vi "SwissSPAD Live_Recording Message.vi"(8 "error in (no error)":errorcluster, 11 "SwissSPAD Live Internal Variables":T1={"okCFrontPanelDevices Refnum"=refnum, "Bottom Device Refnum"=refnum, "Display Image"=refnum, "# Live Images"=0, "relative s"=0.0, "# Image Sets"=0, "Message"="", "Current Image Set"=0, "# Datasets in Series"=0, "Current Dataset"=0, "Live Mode"=FALSE, "Recording Mode"=FALSE, "Record Button"=refnum, "\nLive Button"=refnum, "SwissSPAD Live Gate Image Data Q Name"="SS2 Live Gate Data Q", "Discard First Image"=FALSE, "Image Information"={"Save ROI Only"=FALSE, "Left"=0, "Top"=0, "Right"=0, "Bottom"=0, "Use Current ROI"=FALSE}, "Image Binning Options"={"Use Image Binning"=FALSE, "X Bin"=1, "Y Bin"=1}, "Bottom FPGA Serial Number"="", "Detector PCB Version"=enum."SS2 PCB1", "# Acquisitions"=1, "10 bits"=FALSE, "Top FPGA Serial Number"="", "Top Device Refnum"=refnum} {"# Acquisitions" min=1; "Image Binning Options"."Y Bin" min=1; "Image Binning Options"."X Bin" min=1}) -> (0 "error out":errorcluster, 1 "Current Dataset Recording Completed?":bool, 2 "Message":string, 3 "SwissSPAD Live Internal Variables":T1={"okCFrontPanelDevices Refnum"=refnum, "Bottom Device Refnum"=refnum, "Display Image"=refnum, "# Live Images"=0, "relative s"=0.0, "# Image Sets"=0, "Message"="", "Current Image Set"=0, "# Datasets in Series"=0, "Current Dataset"=0, "Live Mode"=FALSE, "Recording Mode"=FALSE, "Record Button"=refnum, "\nLive Button"=refnum, "SwissSPAD Live Gate Image Data Q Name"="SS2 Live Gate Data Q", "Discard First Image"=FALSE, "Image Information"={"Save ROI Only"=FALSE, "Left"=0, "Top"=0, "Right"=0, "Bottom"=0, "Use Current ROI"=FALSE}, "Image Binning Options"={"Use Image Binning"=FALSE, "X Bin"=1, "Y Bin"=1}, "Bottom FPGA Serial Number"="", "Detector PCB Version"=enum."SS2 PCB1", "# Acquisitions"=1, "10 bits"=FALSE, "Top FPGA Serial Number"="", "Top Device Refnum"=refnum} {"# Acquisitions" min=1; "Image Binning Options"."Y Bin" min=1; "Image Binning Options"."X Bin" min=1}, 4 "Dataset Series Completed?":bool)   [LabVIEW 2021]
uses:
  SwissSPAD Live_Internal Variables.ctl
  D:/UCLA Thinkpad Google Drive/LabVIEW 2021 SP1/builds/SwissSPAD Live Distribution/Opal Kelly/C# Wrapper/v5.0.2/libFrontPanel-csharp.dll
  Opal Kelly/C# Wrapper/v5.0.2/libFrontPanel-csharp.dll
  <vilib>/vision/Image Controls.llb/IMAQ Image.ctl
  SwissSPAD Live_Image ROI Information.ctl
  Phasor/Image Binning Options.ctl
  SwissSPAD Live_SSx PCB Version.ctl
  Sound/System Sounds List.ctl
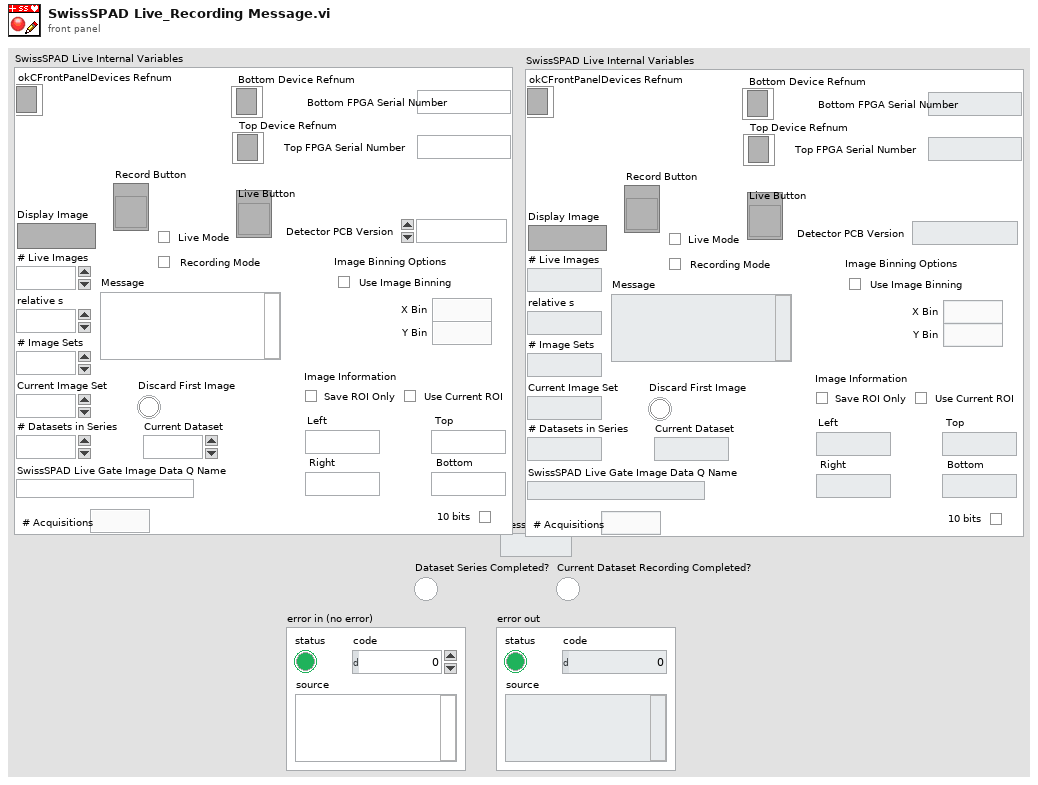
[diagram p1: front panel]
types:
  T1 = typedef "SwissSPAD Live_Internal Variables.ctl" = cluster{"okCFrontPanelDevices Refnum":refnum<k24>, "Bottom Device Refnum":refnum<k24>, "Display Image":T2, "# Live Images":i32, "relative s":dbl, "# Image Sets":i32, "Message":string, "Current Image Set":i32, "# Datasets in Series":i32, "Current Dataset":i32, "Live Mode":bool, "Recording Mode":bool, "Record Button":refnum<vi>, "\nLive Button":refnum<vi>, "SwissSPAD Live Gate Image Data Q Name":string, "Discard First Image":bool, "Image Information":T3, "Image Binning Options":T4, "Bottom FPGA Serial Number":string, "Detector PCB Version":T5, "# Acquisitions":u32, "10 bits":bool, "Top FPGA Serial Number":string, "Top Device Refnum":refnum<k24>}
  T2 = typedef "IMAQ Image.ctl" = refnum<image>
  T3 = typedef "SwissSPAD Live_Image ROI Information.ctl" = cluster{"Save ROI Only":bool, "Left":u16, "Top":u16, "Right":u16, "Bottom":u16, "Use Current ROI":bool}
  T4 = typedef "Image Binning Options.ctl" = cluster{"Use Image Binning":bool, "X Bin":i32, "Y Bin":i32}
  T5 = typedef "SwissSPAD Live_SSx PCB Version.ctl" = enum16{"unknown", "SS2 PCB1", "SS2 PCB2", "SS3 PCB1"}
  T6 = typedef "System Sounds List.ctl" = enum16{"Alarm01", "Alarm02", "Alarm03", "Alarm04", "Alarm05", "Alarm06", "Alarm07", "Alarm08", "Alarm09", "Alarm10", "chimes", "chord", "ding", "notify", "recycle", "Ring01", "Ring02", "Ring03", "Ring04", "Ring05", "Ring06", "Ring07", "Ring08", "Ring09", "Ring10", "ringout", "Speech Off", "Speech On", "Speech Sleep", "tada", "Windows Background", "Windows Balloon", "Windows Battery Critical", "Windows Battery Low", "Windows Critical Stop", "Windows Default", "Windows Ding", "Windows Error", "Windows Exclamation", "Windows Feed Discovered", "Windows Foreground", "Windows Hardware Fail", "Windows Hardware Insert", "Windows Hardware Remove", "Windows Information Bar", "Windows Logoff Sound", "Windows Logon", "Windows Menu Command", "Windows Message Nudge", "Windows Minimize", "Windows Navigation Start", "Windows Notify Calendar", "Windows Notify Email", "Windows Notify Messaging", "Windows Notify System Generic", "Windows Notify", "Windows Pop-up Blocked", "Windows Print complete", "Windows Proximity Connection", "Windows Proximity Notification", "Windows Recycle", "Windows Restore", "Windows Ringin", "Windows Ringout", "Windows Shutdown", "Windows Startup", "Windows Unlock", "Windows User Account Control"}
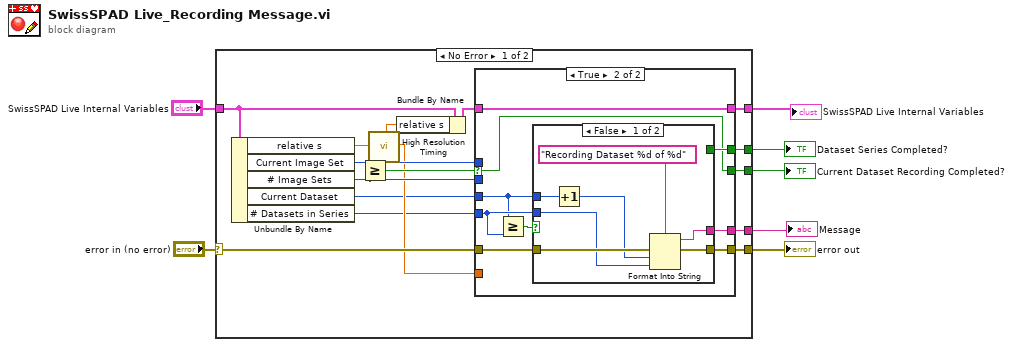
[diagram p0: block diagram]
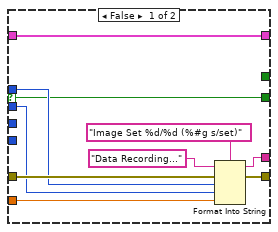
[diagram p2: hidden frame]
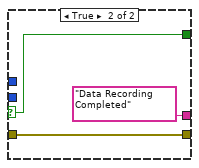
[diagram p3: hidden frame]
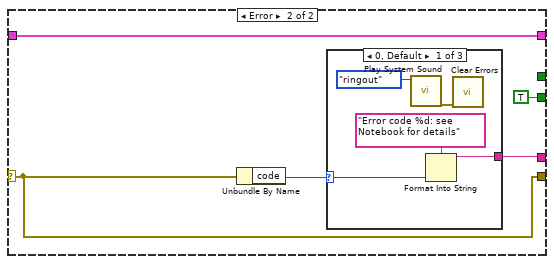
[diagram p4: hidden frame]
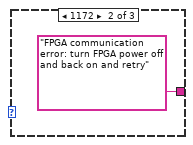
[diagram p5: hidden frame]
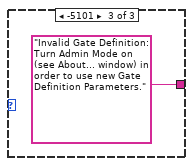
[diagram p6: hidden frame]
diagram:
  n1 = case shown="No Error" "error in (no error)" {
    selector: "error in (no error)" -> [w22 w55]
    tunnel: [w23 w55] -> w7
    tunnel: [w21 w56] -> w5
    tunnel: "SwissSPAD Live Internal Variables" -> [w20 w54]
    tunnel: [w9 w54] -> w3
    tunnel: [w11 TRUE] -> w2
    tunnel: [w8 _] -> w1
    frame No Error {
      n2 = Unbundle By Name(w20) -> ("relative s"=w16:dbl, "Current Image Set"=w18:i32, "# Image Sets"=w17:i32, "Current Dataset"=w13:i32, "# Datasets in Series"=w14:i32)
      n3 = Greater Or Equal?(x=w18, y=w17) -> (x >= y?=w19:bool)
      n4 = call "High Resolution Timing.vi"("relative seconds (NaN)"=w16) -> ("relative seconds"=w12:dbl, "elapsed (relative) seconds"=w15:dbl)  [unwired: 16 in, 1 out]
      n5 = Bundle By Name(cluster=w20, "relative s"=w12) -> (w10:T1)
      n6 = case shown="True" w19 {
        selector: w19 -> [w25 w34]
        tunnel: [w32 w41] -> w23
        tunnel: w22 -> [w31 w42]
        tunnel: [w30 w40] -> w21
        tunnel: w18 -> [w27 _]
        tunnel: w17 -> [w28 _]
        tunnel: w15 -> [w26 _]
        tunnel: w14 -> [_ w38]
        tunnel: w13 -> [_ w35]
        tunnel: [w25 w34] -> w11
        tunnel: w10 -> [w24 w36]
        tunnel: [w24 w36] -> w9
        tunnel: [_ w37] -> w8
        frame False {
          n7 = Format Into String(format string="Image Set %d/%d (%#g s/set)", initial string="Data Recording..." ("Message"), error in=w31, w27, w28, w26) -> (resulting string=w30:string, error out=w32:errorcluster)
        }
        frame True {
          n8 = Greater Or Equal?(x=w35, y=w38) -> (x >= y?=w39:bool)
          n9 = case shown="False" w39 {
            selector: w39 -> [_ w50]
            tunnel: w42 -> [w49 w51]
            tunnel: [w48 w51] -> w41
            tunnel: [w47 "Data Recording Completed"] -> w40
            tunnel: w38 -> [w46 _]
            tunnel: [_ w50] -> w37
            tunnel: w35 -> [w44 _]
            frame False {
              n10 = Increment(x=w44) -> (x+1=w43:i32)
              n11 = Format Into String(format string="Recording Dataset %d of %d", error in=w49, w43, w46) -> (resulting string=w47:string, error out=w48:errorcluster)  [unwired: 1 in]
            }
            frame True {
            }
          }
        }
      }
    }
    frame Error {
      n12 = Unbundle By Name(w55) -> ("code"=w57:i32)
      n13 = case shown="0, Default" w57 {
        selector: w57 -> [w61 _ _]
        tunnel: [w62 "FPGA communication error: turn FPGA power off and back on and retry" "Invalid Gate Definition: Turn Admin Mode on (see About... window) in order to use new Gate Definition Parameters."] -> w56
        frame 0, Default {
          n14 = call "Play System Sound.vi"("Windows Sound"=System_Sounds_List."ringout") -> ("Error Out"=w58:errorcluster)  [unwired: 10 in]
          n15 = Format Into String(format string="Error code %d: see Notebook for details", w61) -> (resulting string=w62:string)  [unwired: 2 in, 1 out]
          n16 = call <vilib>:"Clear Errors.vi"("error in (no error)"=w58) -> ()  [unwired: 5 in, 2 out]
        }
        frame 1172 {
        }
        frame -5101 {
        }
      }
    }
  }
  "error out" <- w7
  "Message" <- w5
  "SwissSPAD Live Internal Variables" <- w3
  "Current Dataset Recording Completed?" <- w2
  "Dataset Series Completed?" <- w1
